vi "Init Tx Conversion Resources.vi"(8 "error in (no error)":errorcluster, 11 "Tx Loop Data":T1) -> (0 "error out":errorcluster, 3 "Tx Loop Data out":T1)   [LabVIEW 2016, in "UDP-Custom-Device Engine.lvlib"]
uses:
  UDP-Custom-Device Engine.lvlib
  Tx Loop Data.ctl
  <vilib>/NI Veristand/VeriStand Data/Library/Byte Buffer/Byte Buffer.lvclass
  <vilib>/NI/NIVS Inline Async API/_Data Access Engine/Data Access Engine/Types/Read.DVR.ctl
  <vilib>/NI/NIVS Inline Async API/_Data Access Engine/Access Type Classes/Read/Read.lvclass
  <vilib>/NI Veristand/VeriStand Data/Library/Typedefs/Typedefs.Data Types.ctl
  Data Conversion Config.ctl
  <vilib>/NI Veristand/VeriStand Data/Library/Byte Buffer/Byte Buffer.Mapping.ctl
  <vilib>/NI Veristand/VeriStand Data/Library/Byte Buffer/Byte Buffer.Mapping.Create (Channel Pointer).vi
  <vilib>/NI Veristand/VeriStand Data/Library/Utilities/Utilities.Sizeof.Array.vi
  <vilib>/NI Veristand/VeriStand Data/Library/Utilities/Utilities.Sizeof.Scalar.vi
  <vilib>/NI Veristand/VeriStand Data/Library/VeriStand Data.lvlib
  <vilib>/NI/NIVS Inline Async API/_Data Access Engine/Data Access Engine/Data Access Engine.lvclass
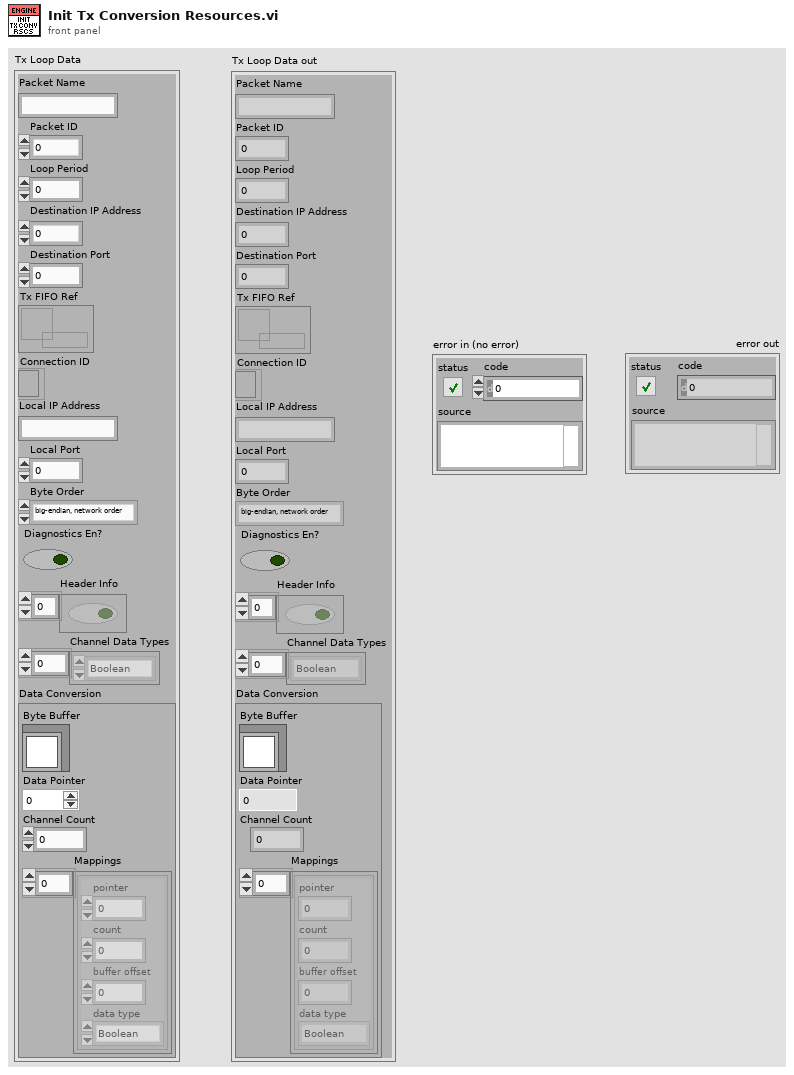
[diagram p1: front panel]
types:
  T1 = typedef "UDP-Custom-Device Engine.lvlib/Tx Loop Data.ctl" = cluster{"Packet Name":string, "Packet ID":i32, "Loop Period":u32, "Destination IP Address":u32, "Destination Port":u16, "Tx FIFO Ref":T2, "Connection ID":refnum<k16>, "Local IP Address":string, "Local Port":i32, "Byte Order":enum16{"big-endian, network order", "native, host order", "little-endian"}, "Diagnostics En?":bool, "Header Info":bool[], "Channel Data Types":T3[], "Data Conversion":T4}
  T2 = typedef "Data Access Engine.lvlib/Data Access Engine.lvclass/Read.DVR.ctl" = refnum<data-value>
  T3 = typedef "VeriStand Data.lvlib/Typedefs.Data Types.ctl" = enum16{"Boolean", "Single", "Double", "I8", "I16", "I32", "I64", "U8", "U16", "U32", "U64"}
  T4 = typedef "UDP-Custom-Device Engine.lvlib/Data Conversion Config.ctl" = cluster{"Byte Buffer":refnum<class "Byte Buffer.lvclass">, "Data Pointer":u64, "Channel Count":i32, "Mappings":T5[]}
  T5 = typedef "VeriStand Data.lvlib/Byte Buffer.lvclass/Byte Buffer.Mapping.ctl" = cluster{"pointer":u64, "count":i32, "buffer offset":i32, "data type":T3}
  T6 = enum16{"big-endian, network order", "native, host order", "little-endian"}
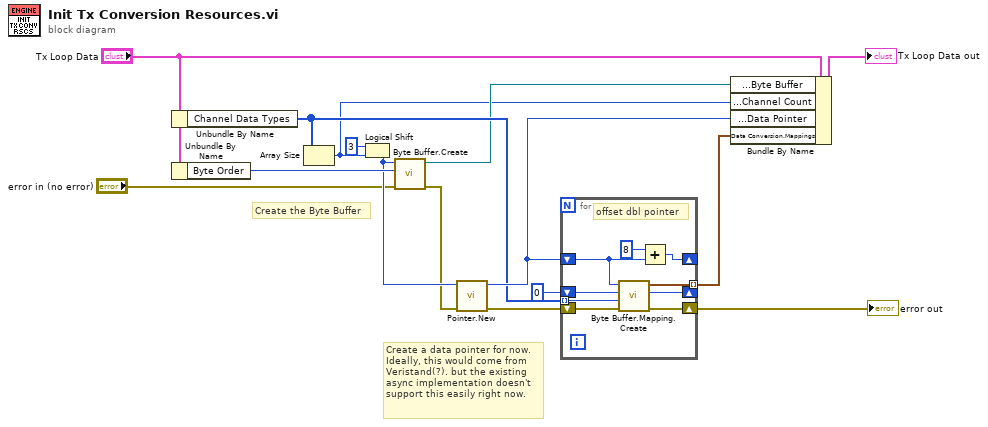
[diagram p0: block diagram]
diagram:
  # "Create the Byte Buffer"
  # "Create a data pointer for now.\nIdeally, this would come from\nVeristand(?). but the existing\nasync implementation doesn't\nsupport this easily right now."
  n1 = Unbundle By Name("Tx Loop Data") -> ("Channel Data Types"=w9:T3[])
  n2 = Unbundle By Name("Tx Loop Data") -> ("Byte Order"=w14:T6)
  n3 = Array Size(array=w9) -> (size(s)=w7:i32)
  n4 = Logical Shift(y=i16 3, x=w7) -> (x << y=w4:i32)
  n5 = call <vilib>:"Byte Buffer.Create.vi"("error in (no error)"="error in (no error)", "byte order (big-endian)"=w14, "size"=w4) -> ("error out"=w1:errorcluster, "Byte Buffer"=w8:refnum<class "Byte Buffer.lvclass">)  [unwired: 7 in]
  n6 = call <vilib>:"Pointer.New.vi"("error in (no error)"=w1, "size in bytes"=w4) -> ("error out"=w11:errorcluster, "pointer"=w12:u64)  [unwired: 8 in]
  n7 = for {
    tunnel: [w24] -> w13 mode=indexing
    tunnel: w9 -> [w21] mode=indexing
    shift-right: [w22] -> w3
    shift-left: w11 -> [w23]
    shift-right: [w19] -> _
    shift-left: w12 -> [w20]
    shift-right: [w17] -> _
    shift-left: 0 ("new buffer offset") -> [w16]
    # "offset dbl pointer"
    n8 = call-poly <vilib>:"Byte Buffer.Mapping.Create.vi"("error in (no error)"=w23, "data type"=w21, "buffer offset"=w16, "Channel Pointer"=w20) -> ("error out"=w22:errorcluster, "new buffer offset"=w17:i32, "mapping"=w24:T5)  [unwired: 5 in]
    n9 = Add(x=u64 8, y=w20) -> (x+y=w19:u64)
  }
  "error out" <- w3
  n10 = Bundle By Name(cluster="Tx Loop Data", "Data Conversion.Byte Buffer"=w8, "Data Conversion.Channel Count"=w7, "Data Conversion.Data Pointer"=w12, "Data Conversion.Mappings"=w13) -> (→"Tx Loop Data out":T1)
